vi "Mars3D_new.vi"(7 "Statemachine Data IN":T1={"Impulse Positions"=[], "Old Impulse positions for Undo"=[], "No. Imp"=0, "Parameter Time Series"=[], "Parameter Impuls Series"=[], "Experiment Parameters"={"Freq"=0.0, "Vel"=0, "Acc"=0, "Stimulus"=""}, "Autosort File"=refnum, "Data File"={"Data Channels"=[], "Sample Rate"=0, "Channel List"=[]}, "Experiment data path"=path "/Macintosh HD/Users/patrick/Studium/Diploma Thesis/Data Analysis", "Image data path"=path "/Macintosh HD/Users/patrick/Studium/Diploma Thesis/Data Analysis", "LVS data path"=path "/Macintosh HD/Users/patrick/Studium/Diploma Thesis/Data Analysis", "Raw copy path"=path "/Macintosh HD/Users/patrick/Studium/Diploma Thesis/Data Analysis", "filename"="No file selected", "desaccading parameters"={"Tolerance"=0, "Acc Range"=0.0, "Sample Rate"=0, "Impulse Plane 2"=enum."Other", "Impulse dir"=FALSE}, "Experiment Parameters 2"={"Subject"="", "Strain"="", "Rotation plane"="", "Experimenter"="", "Trial"=0.0, "Time"=0.0}, "Excel"={"Excel._Application"=refnum, "Use Excel"=FALSE, "Worksheet SINE"=refnum, "Row SINE"=0, "Worksheet TRANS"=refnum, "Row TRANS"=0}, "Session Config File"=refnum, "Autosort Parameter Set"=1, "EMA Version"="", "desacc "={"Threshold 1 [Acc]"=1617.080808080808, "Threshold 2 [% of TH1]"=67, "tolerance"=5, "Search WD "=0.19090909090909092, " always use TH2"=TRUE, "Range"=3.2323232323232323, "Max time"=200.0, "Min time"=20.0, "Velocity Threshold"=67}, "Cycle Nr for Saccades"={"POS"=0, "NEG"=0}, "Undo Counter"=0, "History Length"=0, "Redo Counter"=0, "Histpry Position"=0, "Raw Data File"={"Data Channels"=[], "Sample Rate"=0, "Channel List"=[]}, "calibration name"="No file selected"} {"Parameter Time Series"."time offset" format="%.3f"; "Parameter Time Series"."Gain" format="%.1f"; "Parameter Time Series"."Offset" format="%.1f"; "Parameter Time Series"."List 1" items=["Motor-Pos", "Motor-Vel", "Lx Position-in-Head", "Ly Position-in-Head", "Lz Position-in-Head", "Lx Velocity-in-Head", "Ly Velocity-in-Head", "Lz Velocity-in-Head", "Ll Velocity-in-Head", "Lr Velocity-in-Head", "Lx Accel-in-Head", "Ly Accel-in-Head", "Lz Accel-in-Head", "Rx Position-in-Head", "Ry Position-in-Head", "Rz Position-in-Head", "Rx Velocity-in-Head", "Ry Velocity-in-Head", "Rz Velocity-in-Head", "Rl Velocity-in-Head", "Rr Velocity-in-Head", "Rx Accel-in-Head", "Ry Accel-in-Head", "Rz Accel-in-Head", "Global Trigger", "", "", ""]; "Parameter Impuls Series"."Gain" format="%.1f"; "Parameter Impuls Series"."Offset" format="%.1f"}, 10 "File":path) -> (1 "stop 3":bool, 5 "Statemachine Data OUT":T1={"Impulse Positions"=[], "Old Impulse positions for Undo"=[], "No. Imp"=0, "Parameter Time Series"=[], "Parameter Impuls Series"=[], "Experiment Parameters"={"Freq"=0.0, "Vel"=0, "Acc"=0, "Stimulus"=""}, "Autosort File"=refnum, "Data File"={"Data Channels"=[], "Sample Rate"=0, "Channel List"=[]}, "Experiment data path"=path "/Macintosh HD/Users/patrick/Studium/Diploma Thesis/Data Analysis", "Image data path"=path "/Macintosh HD/Users/patrick/Studium/Diploma Thesis/Data Analysis", "LVS data path"=path "/Macintosh HD/Users/patrick/Studium/Diploma Thesis/Data Analysis", "Raw copy path"=path "/Macintosh HD/Users/patrick/Studium/Diploma Thesis/Data Analysis", "filename"="No file selected", "desaccading parameters"={"Tolerance"=0, "Acc Range"=0.0, "Sample Rate"=0, "Impulse Plane 2"=enum."Other", "Impulse dir"=FALSE}, "Experiment Parameters 2"={"Subject"="", "Strain"="", "Rotation plane"="", "Experimenter"="", "Trial"=0.0, "Time"=0.0}, "Excel"={"Excel._Application"=refnum, "Use Excel"=FALSE, "Worksheet SINE"=refnum, "Row SINE"=0, "Worksheet TRANS"=refnum, "Row TRANS"=0}, "Session Config File"=refnum, "Autosort Parameter Set"=1, "EMA Version"="", "desacc "={"Threshold 1 [Acc]"=1617.080808080808, "Threshold 2 [% of TH1]"=67, "tolerance"=5, "Search WD "=0.19090909090909092, " always use TH2"=TRUE, "Range"=3.2323232323232323, "Max time"=200.0, "Min time"=20.0, "Velocity Threshold"=67}, "Cycle Nr for Saccades"={"POS"=0, "NEG"=0}, "Undo Counter"=0, "History Length"=0, "Redo Counter"=0, "Histpry Position"=0, "Raw Data File"={"Data Channels"=[], "Sample Rate"=0, "Channel List"=[]}, "calibration name"="No file selected"} {"Parameter Time Series"."time offset" format="%.3f"; "Parameter Time Series"."Gain" format="%.1f"; "Parameter Time Series"."Offset" format="%.1f"; "Parameter Time Series"."List 1" items=["Motor-Pos", "Motor-Vel", "Lx Position-in-Head", "Ly Position-in-Head", "Lz Position-in-Head", "Lx Velocity-in-Head", "Ly Velocity-in-Head", "Lz Velocity-in-Head", "Ll Velocity-in-Head", "Lr Velocity-in-Head", "Lx Accel-in-Head", "Ly Accel-in-Head", "Lz Accel-in-Head", "Rx Position-in-Head", "Ry Position-in-Head", "Rz Position-in-Head", "Rx Velocity-in-Head", "Ry Velocity-in-Head", "Rz Velocity-in-Head", "Rl Velocity-in-Head", "Rr Velocity-in-Head", "Rx Accel-in-Head", "Ry Accel-in-Head", "Rz Accel-in-Head", "Global Trigger", "", "", ""]; "Parameter Impuls Series"."Gain" format="%.1f"; "Parameter Impuls Series"."Offset" format="%.1f"})   [LabVIEW 2016]
uses:
  core/type-defs/TD_Statemachine-Data.ctl
  core/type-defs/TD_Time Series.ctl
  core/type-defs/TD_Impulse Parameter.ctl
  <vilib>/Utility/file.llb/Read From Spreadsheet File (DBL).vi
  tracking algorithmus/3 dot tracker.lvlib
  <vilib>/Analysis/NI_AALPro.lvlib
  core/core.lvlib
panel:
  in  "Savol Filter in percent":dbl=3.0 format="%#_13g"
  in  "stop 2":bool
  in  "VOG system":enum16{"Mouse", "Chinchilla"}(ring)
  in  "Tab Control":T4(tab)
  in  "Savgol":bool
  in  "Right Eye":T5 {"y" format="%.2f"; "z" format="%.2f"; "theta" format="%.2f"; "phi" format="%.2f"; "d" format="%.2f"}
  in  "Left Eye":T5 {"y" format="%.2f"; "z" format="%.2f"; "theta" format="%.2f"; "phi" format="%.2f"; "d" format="%.2f"}
  in  "Position Convention":u16(ring)=1 items=["Fick Angles", "Rotation Vectors"]
  in  "Angles":bool
  in  "Automatic Calibration":bool=TRUE
  in  "Rev Cam?":bool caption="Reverse Camera\nOrientation?"
  in  "Plot Selection":T2=[{"time offset"=0.0, "Offset"=0.0, "Gain"=1.0, "inverse"=FALSE, "filter data"=FALSE, "dots"=FALSE, "interpolate"=FALSE, "List 1"=1, "Color Box"=0, "Boolean"=TRUE}, {"time offset"=0.0, "Offset"=0.0, "Gain"=1.0, "inverse"=FALSE, "filter data"=FALSE, "dots"=FALSE, "interpolate"=FALSE, "List 1"=7, "Color Box"=16860, "Boolean"=TRUE}, {"time offset"=0.0, "Offset"=0.0, "Gain"=1.0, "inverse"=FALSE, "filter data"=FALSE, "dots"=FALSE, "interpolate"=FALSE, "List 1"=18, "Color Box"=16711680, "Boolean"=TRUE}] {"time offset" format="%.3f"; "Gain" format="%.1f"; "Offset" format="%.1f"; "List 1" items=["Motor-Pos", "Motor-Vel", "Lx Position-in-Head", "Ly Position-in-Head", "Lz Position-in-Head", "Lx Velocity-in-Head", "Ly Velocity-in-Head", "Lz Velocity-in-Head", "Ll Velocity-in-Head", "Lr Velocity-in-Head", "Lx Accel-in-Head", "Ly Accel-in-Head", "Lz Accel-in-Head", "Rx Position-in-Head", "Ry Position-in-Head", "Rz Position-in-Head", "Rx Velocity-in-Head", "Ry Velocity-in-Head", "Rz Velocity-in-Head", "Rl Velocity-in-Head", "Rr Velocity-in-Head", "Rx Accel-in-Head", "Ry Accel-in-Head", "Rz Accel-in-Head", "Global Trigger", "Free 1", "Free 2", "Free 3"]}
  in  "Plot Selection 2":T3=[{"Color"=4652800, "Visible"=TRUE, "Channel"=1, "Invert"=FALSE, "Desaccade"=FALSE, "Offset"=0.0, "Gain"=1.0}, {"Color"=16860, "Visible"=TRUE, "Channel"=7, "Invert"=FALSE, "Desaccade"=FALSE, "Offset"=0.0, "Gain"=1.0}, {"Color"=16711680, "Visible"=TRUE, "Channel"=18, "Invert"=FALSE, "Desaccade"=FALSE, "Offset"=0.0, "Gain"=1.0}] {"Gain" format="%.1f"; "Offset" format="%.1f"; "Channel" items=["Motor-Pos", "Motor-Vel", "Lx Position-in-Head", "Ly Position-in-Head", "Lz Position-in-Head", "Lx Velocity-in-Head", "Ly Velocity-in-Head", "Lz Velocity-in-Head", "Ll Velocity-in-Head", "Lr Velocity-in-Head", "Lx Accel-in-Head", "Ly Accel-in-Head", "Lz Accel-in-Head", "Rx Position-in-Head", "Ry Position-in-Head", "Rz Position-in-Head", "Rx Velocity-in-Head", "Ry Velocity-in-Head", "Rz Velocity-in-Head", "Rl Velocity-in-Head", "Rr Velocity-in-Head", "Rx Accel-in-Head", "Ry Accel-in-Head", "Rz Accel-in-Head", "Global Trigger", "Free 1", "Free 2", "Free 3"]}
  in  "Tolerance":i32(slide)=40 step=2 scale=0.0..100.0
  in  "Acc Range":dbl(slide)=3000.0 step=50.0 scale=0.0..30000.0
  in  "Impulse dir":bool
  in  "Impulse Plane 2":T6(ring)=enum."Yaw" caption="Impulse Plane"
  in  "process":bool
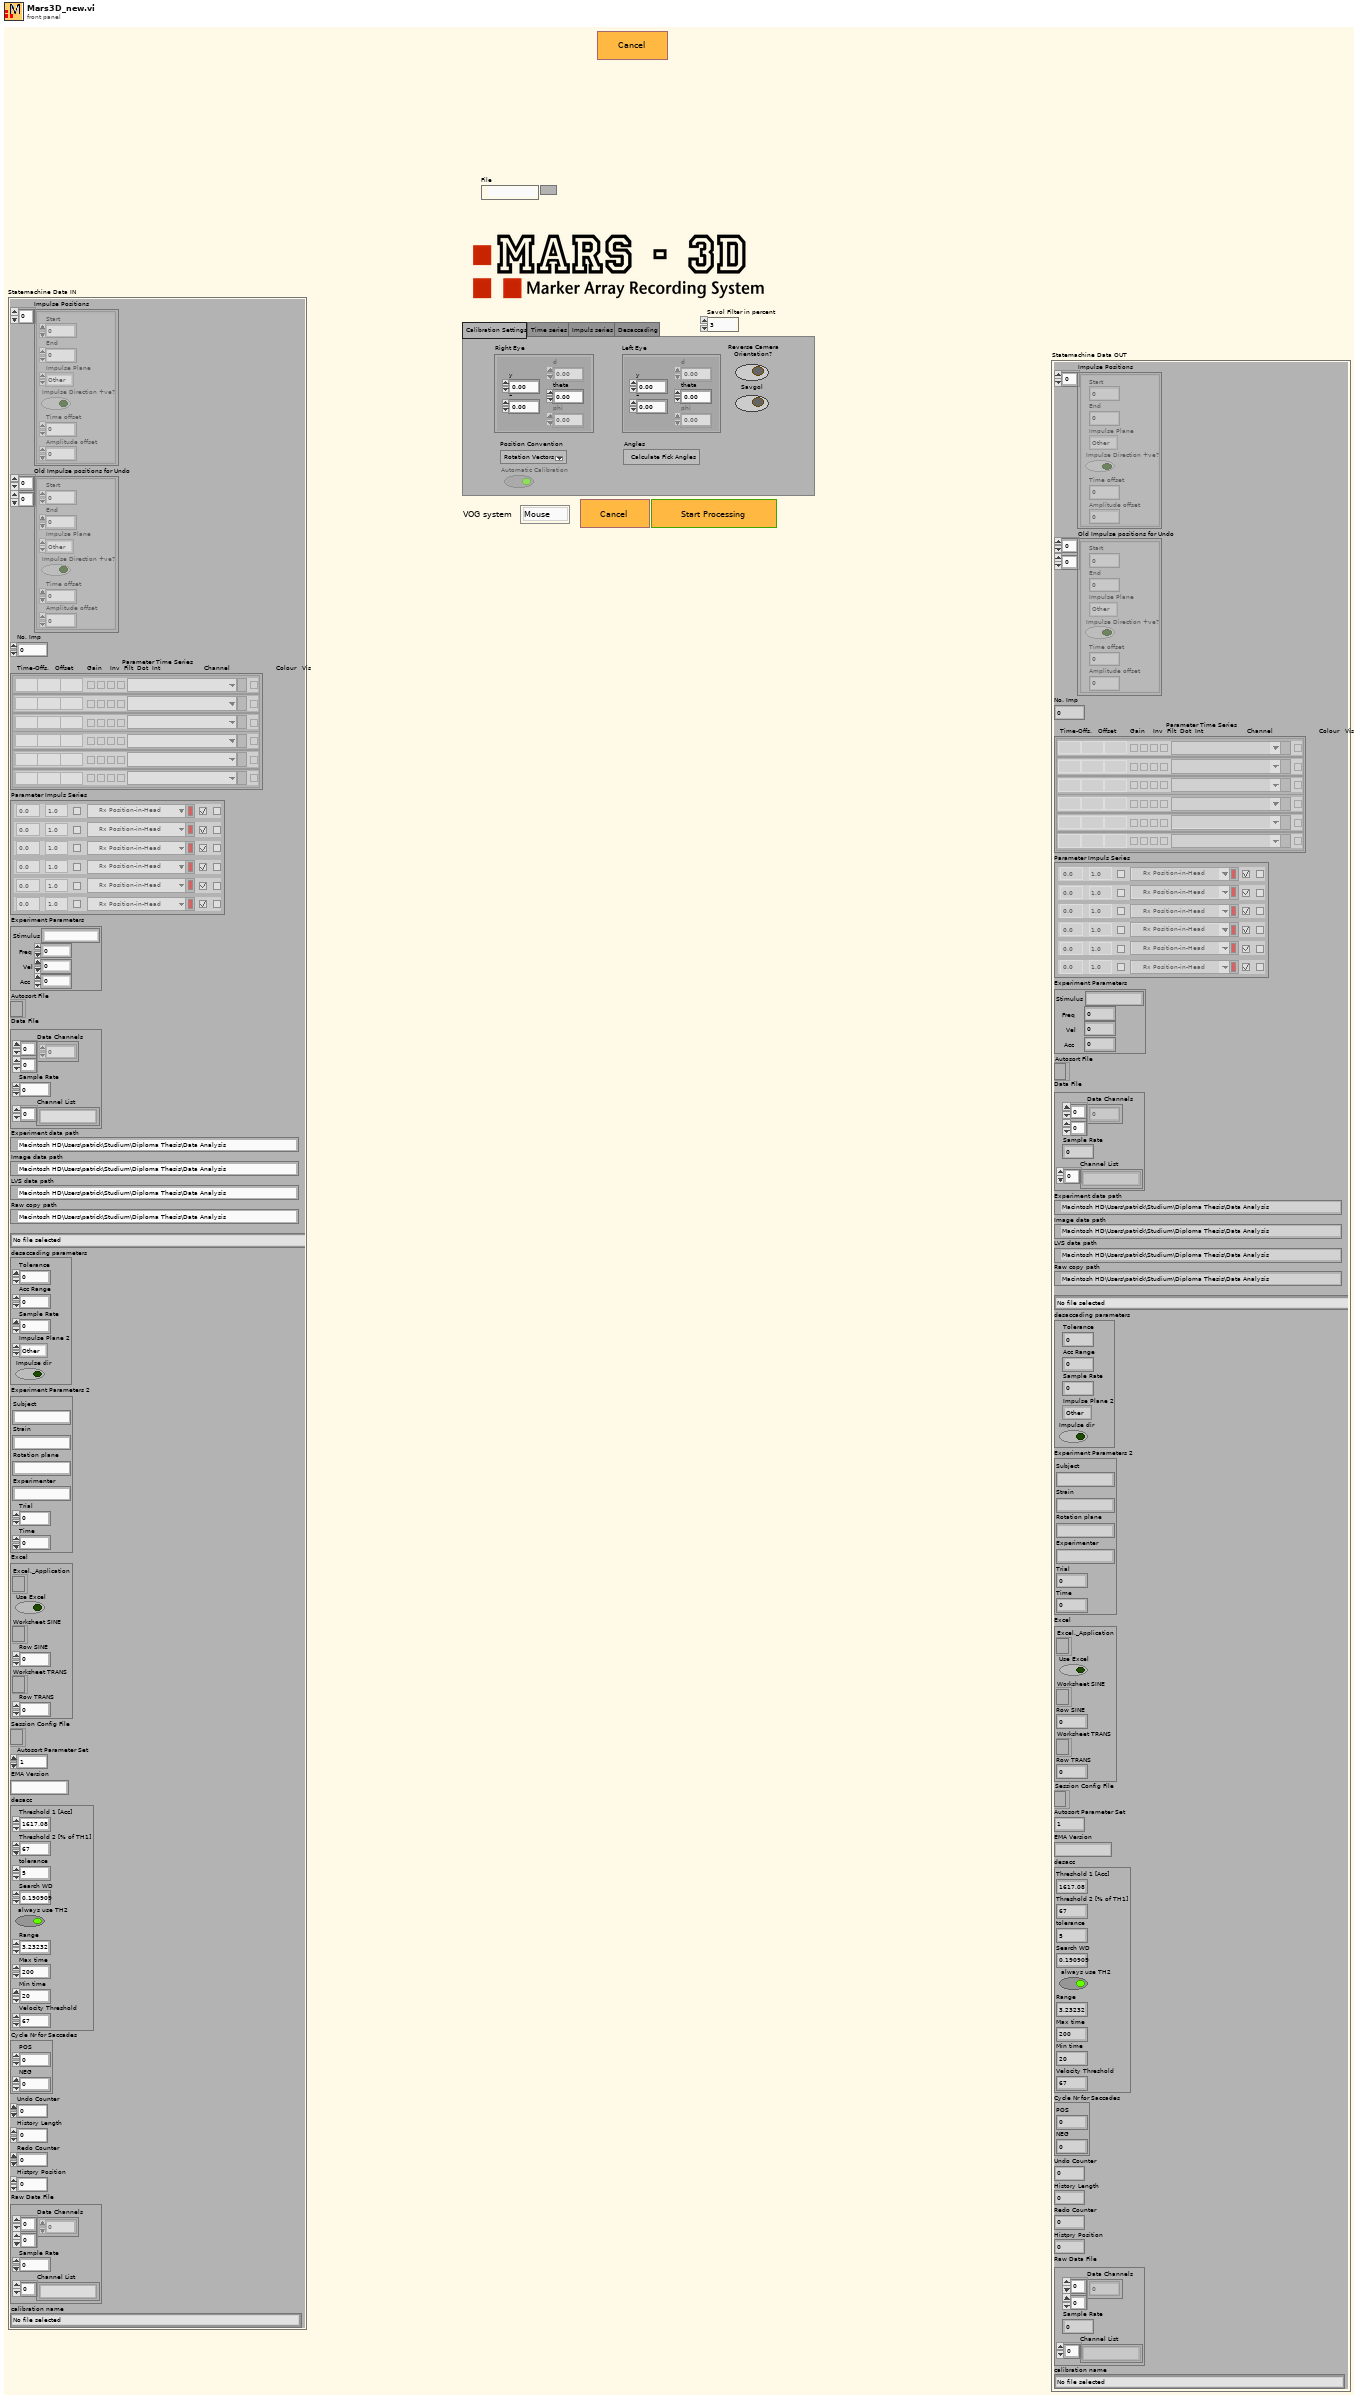
[diagram p1: front panel]
types:
  T1 = typedef "core.lvlib/TD_Statemachine-Data.ctl" = cluster{"Impulse Positions":cluster{"Start":i32, "End":i32, "Impulse Plane":enum16{"Other", "Yaw", "Pitch", "Roll", "LARP", "RALP"}, "Impulse Direction +ve?":bool, "Time offset":i32, "Amplitude offset":dbl}[], "Old Impulse positions for Undo":cluster{"Start":i32, "End":i32, "Impulse Plane":enum16{"Other", "Yaw", "Pitch", "Roll", "LARP", "RALP"}, "Impulse Direction +ve?":bool, "Time offset":i32, "Amplitude offset":dbl}[][], "No. Imp":i32, "Parameter Time Series":T2, "Parameter Impuls Series":T3, "Experiment Parameters":cluster{"Freq":dbl, "Vel":i32, "Acc":i32, "Stimulus":string}, "Autosort File":refnum<file>, "Data File":cluster{"Data Channels":dbl[][], "Sample Rate":i32, "Channel List":string[]}, "Experiment data path":path, "Image data path":path, "LVS data path":path, "Raw copy path":path, "filename":string, "desaccading parameters":cluster{"Tolerance":i32, "Acc Range":dbl, "Sample Rate":i32, "Impulse Plane 2":enum16{"Other", "Yaw", "Pitch", "Roll", "LARP", "RALP"}, "Impulse dir":bool}, "Experiment Parameters 2":cluster{"Subject":string, "Strain":string, "Rotation plane":string, "Experimenter":string, "Trial":dbl, "Time":dbl}, "Excel":cluster{"Excel._Application":refnum<k7>, "Use Excel":bool, "Worksheet SINE":refnum<k7>, "Row SINE":i32, "Worksheet TRANS":refnum<k7>, "Row TRANS":i32}, "Session Config File":refnum<file>, "Autosort Parameter Set":i32, "EMA Version":string, "desacc ":cluster{"Threshold 1 [Acc]":dbl, "Threshold 2 [% of TH1]":i32, "tolerance":i32, "Search WD ":dbl, " always use TH2":bool, "Range":dbl, "Max time":dbl, "Min time":dbl, "Velocity Threshold":i32}, "Cycle Nr for Saccades":cluster{"POS":i32, "NEG":i32}, "Undo Counter":i32, "History Length":i32, "Redo Counter":i32, "Histpry Position":i32, "Raw Data File":cluster{"Data Channels":dbl[][], "Sample Rate":i32, "Channel List":string[]}, "calibration name":string}
  T2 = typedef "core.lvlib/TD_Time Series.ctl" = cluster{"time offset":dbl, "Offset":dbl, "Gain":dbl, "inverse":bool, "filter data":bool, "dots":bool, "interpolate":bool, "List 1":u16, "Color Box":u32, "Boolean":bool}[]
  T3 = typedef "core.lvlib/TD_Impulse Parameter.ctl" = cluster{"Color":u32, "Visible":bool, "Channel":u16, "Invert":bool, "Desaccade":bool, "Offset":dbl, "Gain":dbl}[]
  T4 = enum32{"Calibration Settings", "Time series", "Impuls series", "Desaccading"}
  T5 = cluster{"d":dbl, "phi":dbl, "theta":dbl, "z":dbl, "y":dbl}
  T6 = enum16{"Other", "Yaw", "Pitch", "Roll", "LARP", "RALP"}
  T7 = cluster{"Tolerance":i32, "Acc Range":dbl, "Sample Rate":i32, "Impulse Plane 2":enum16{"Other", "Yaw", "Pitch", "Roll", "LARP", "RALP"}, "Impulse dir":bool}
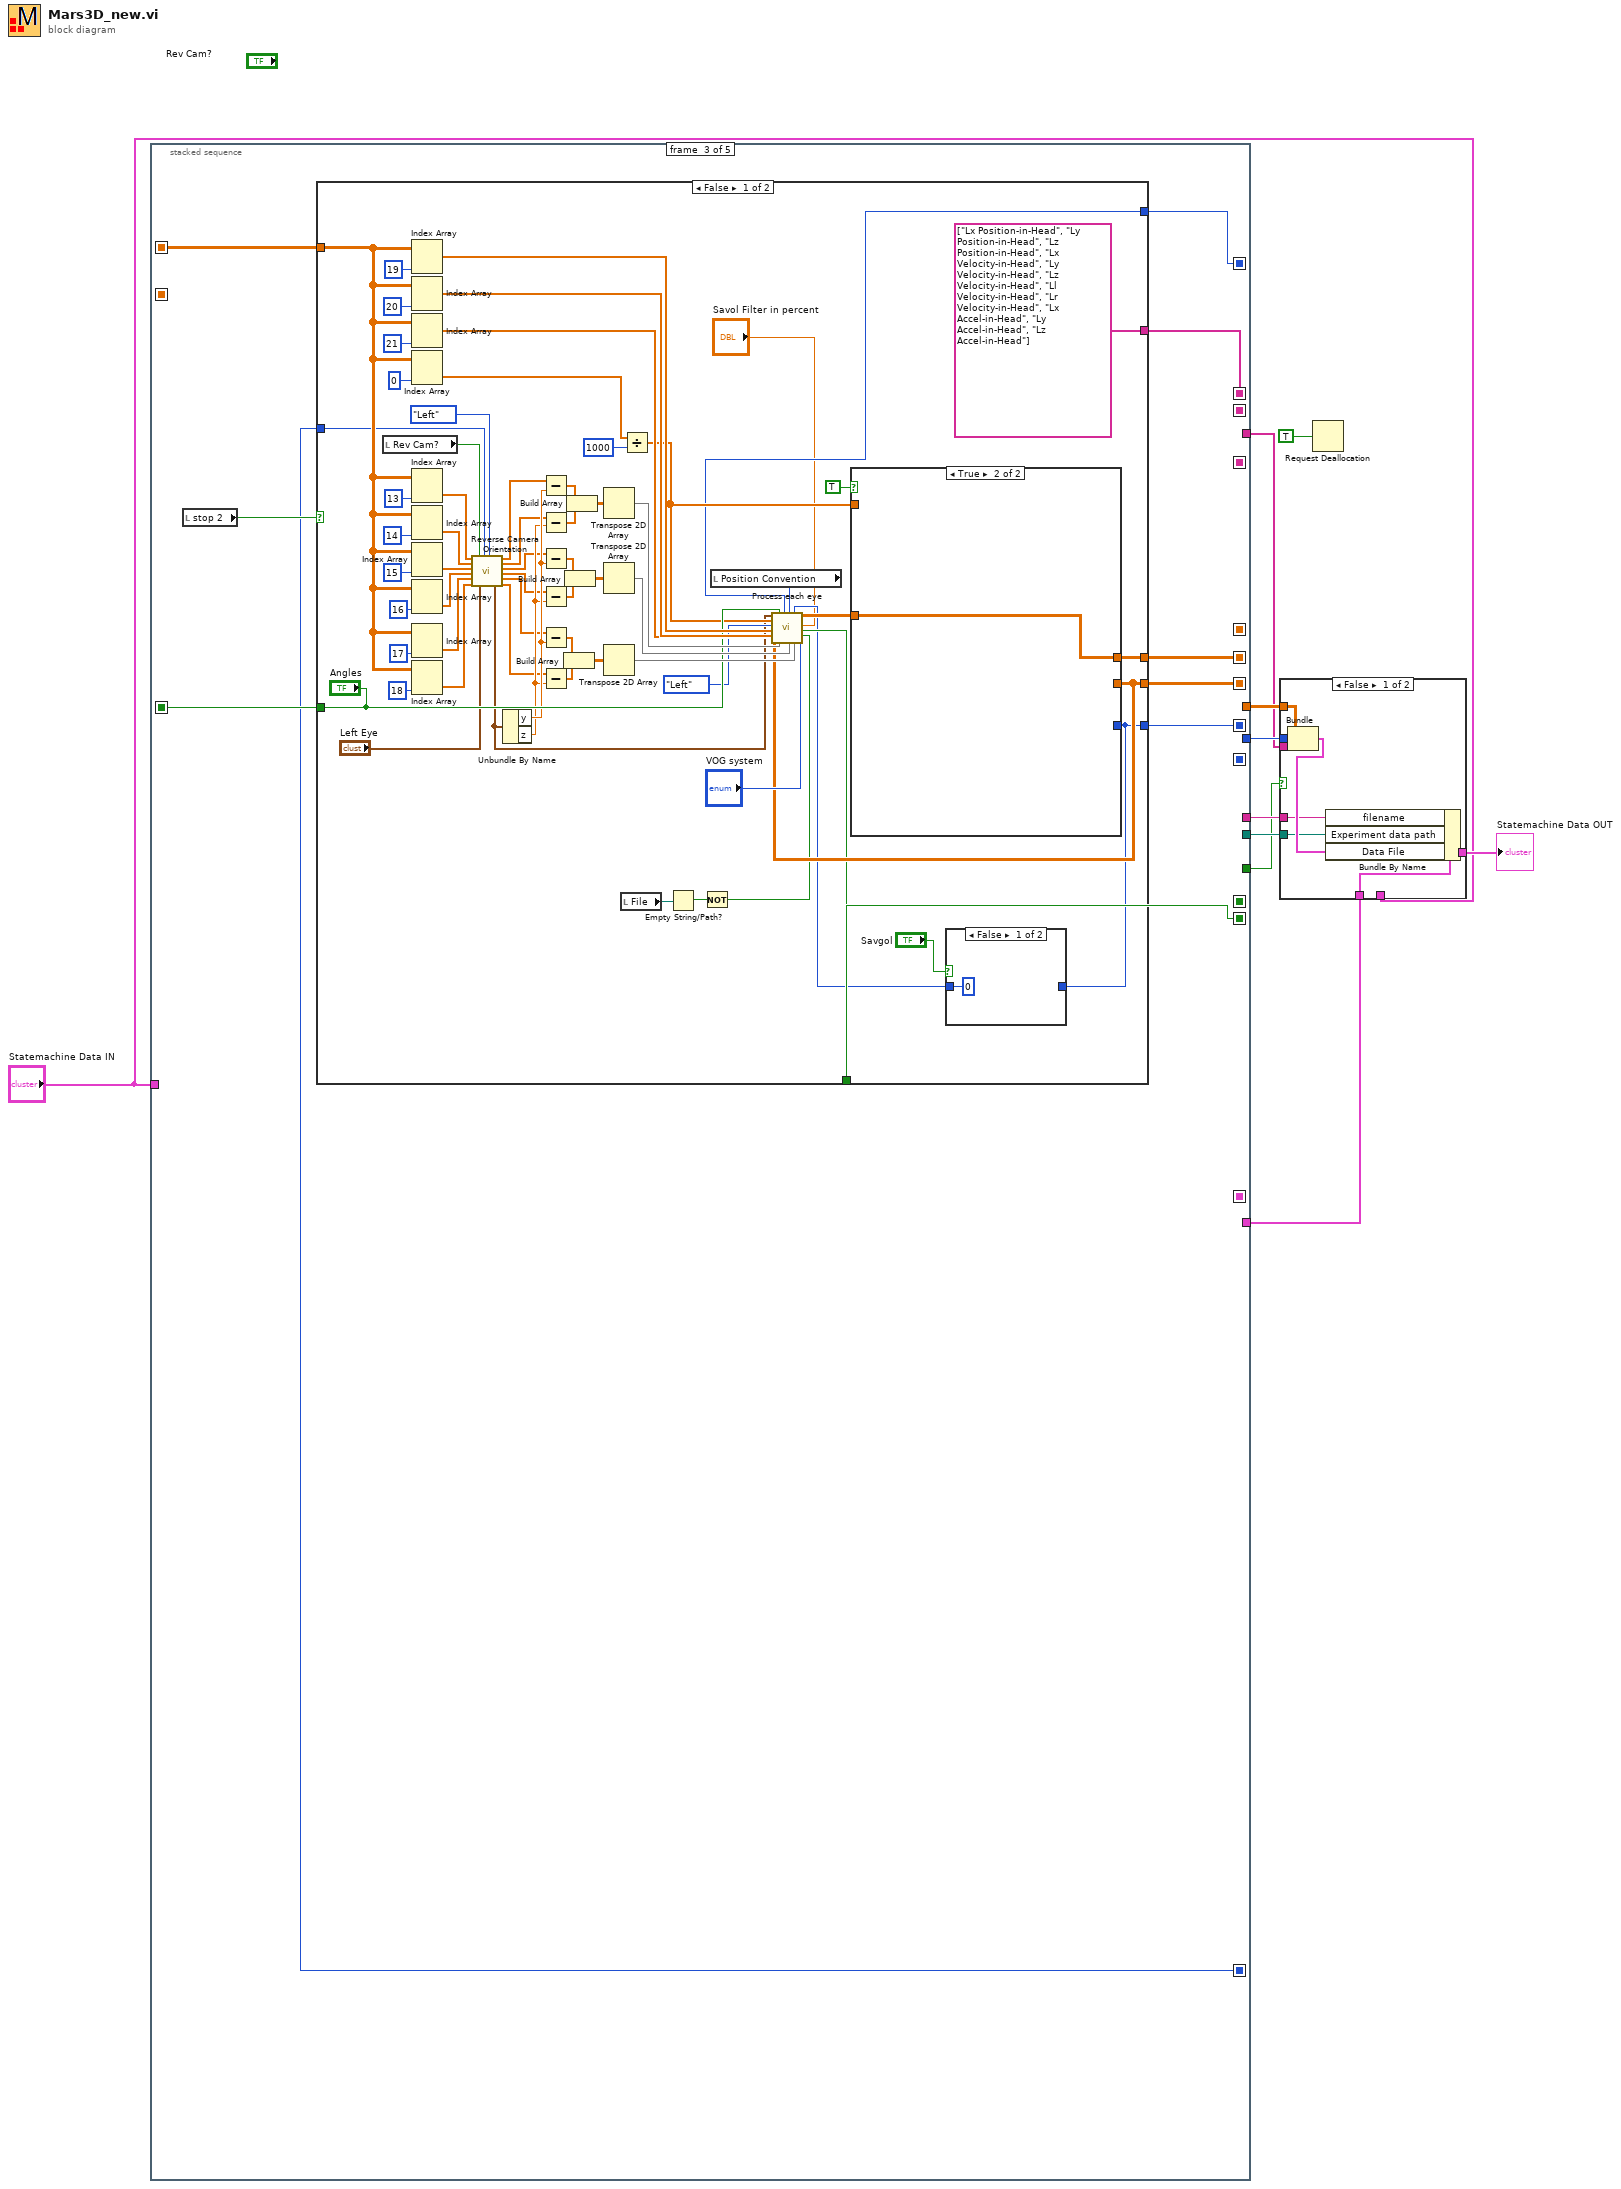
[diagram p0: block diagram]
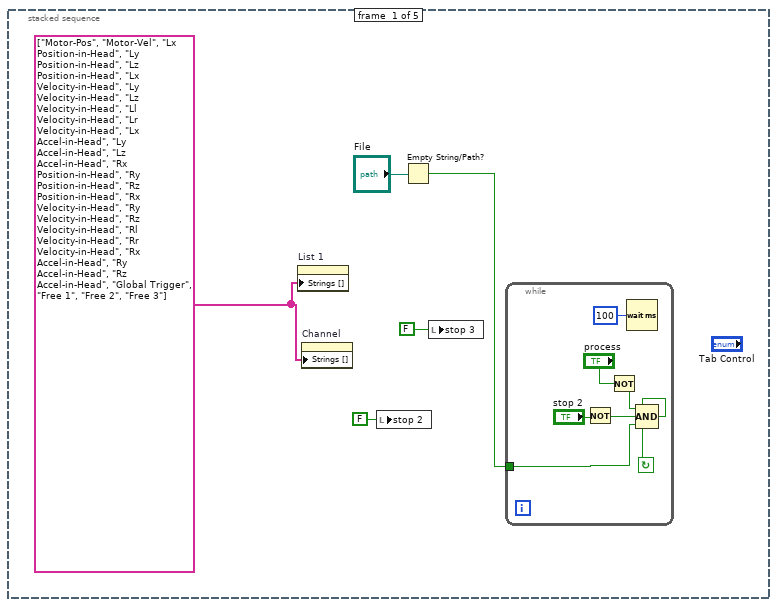
[diagram p3: hidden frame]
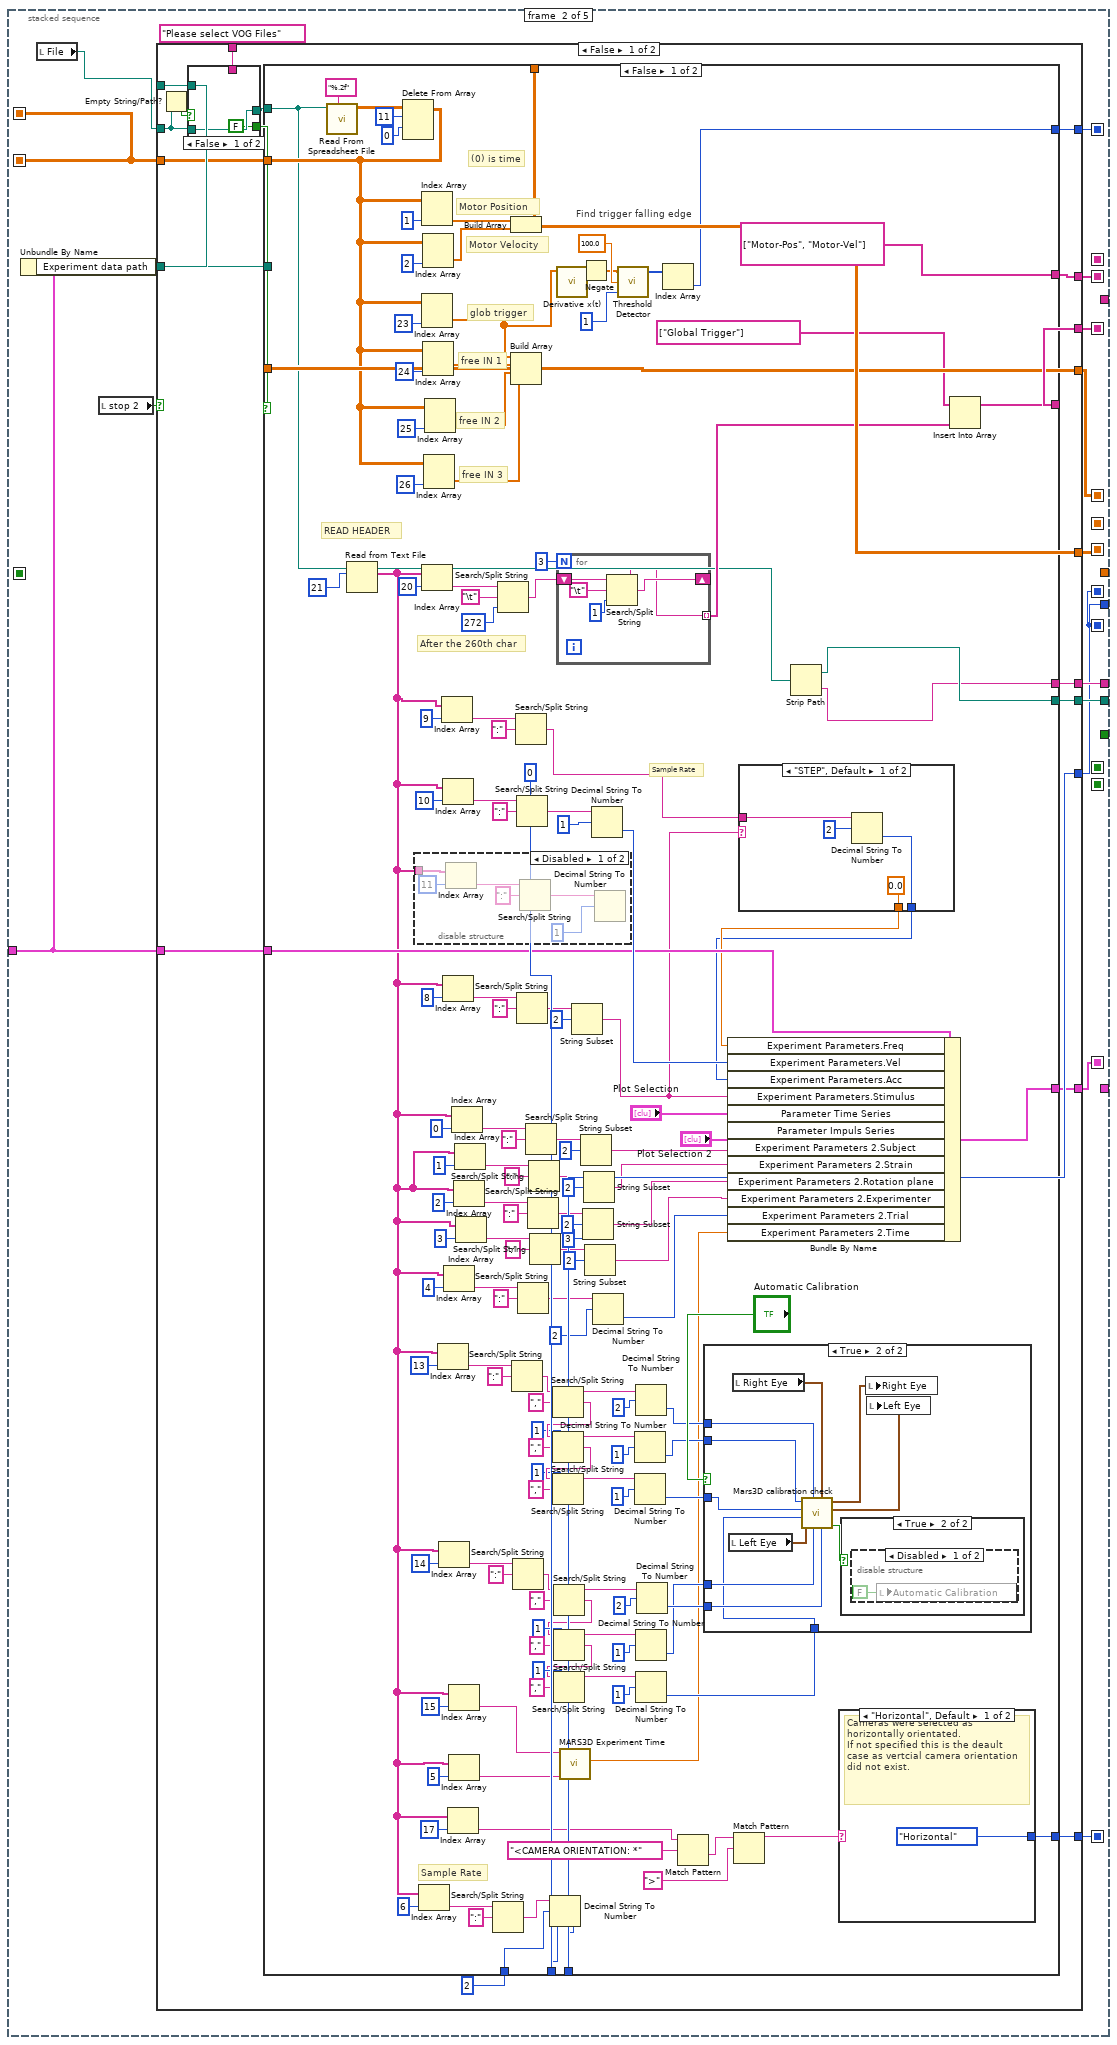
[diagram p4: hidden frame]
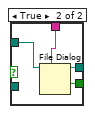
[diagram p5: hidden frame]
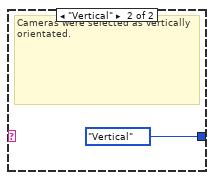
[diagram p6: hidden frame]
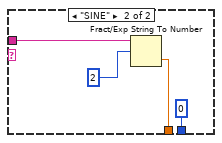
[diagram p7: hidden frame]
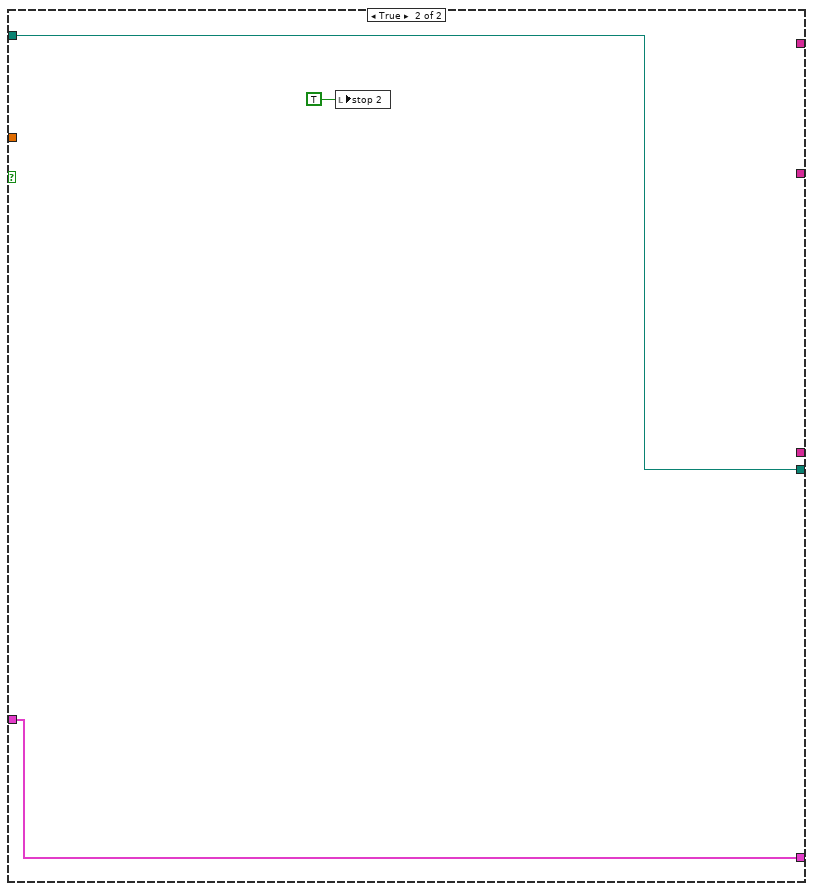
[diagram p12: hidden frame]
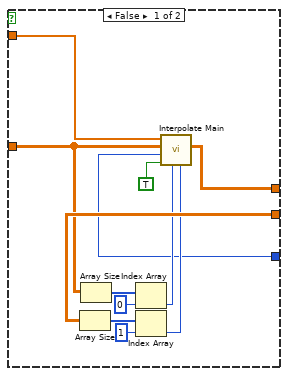
[diagram p15: hidden frame]
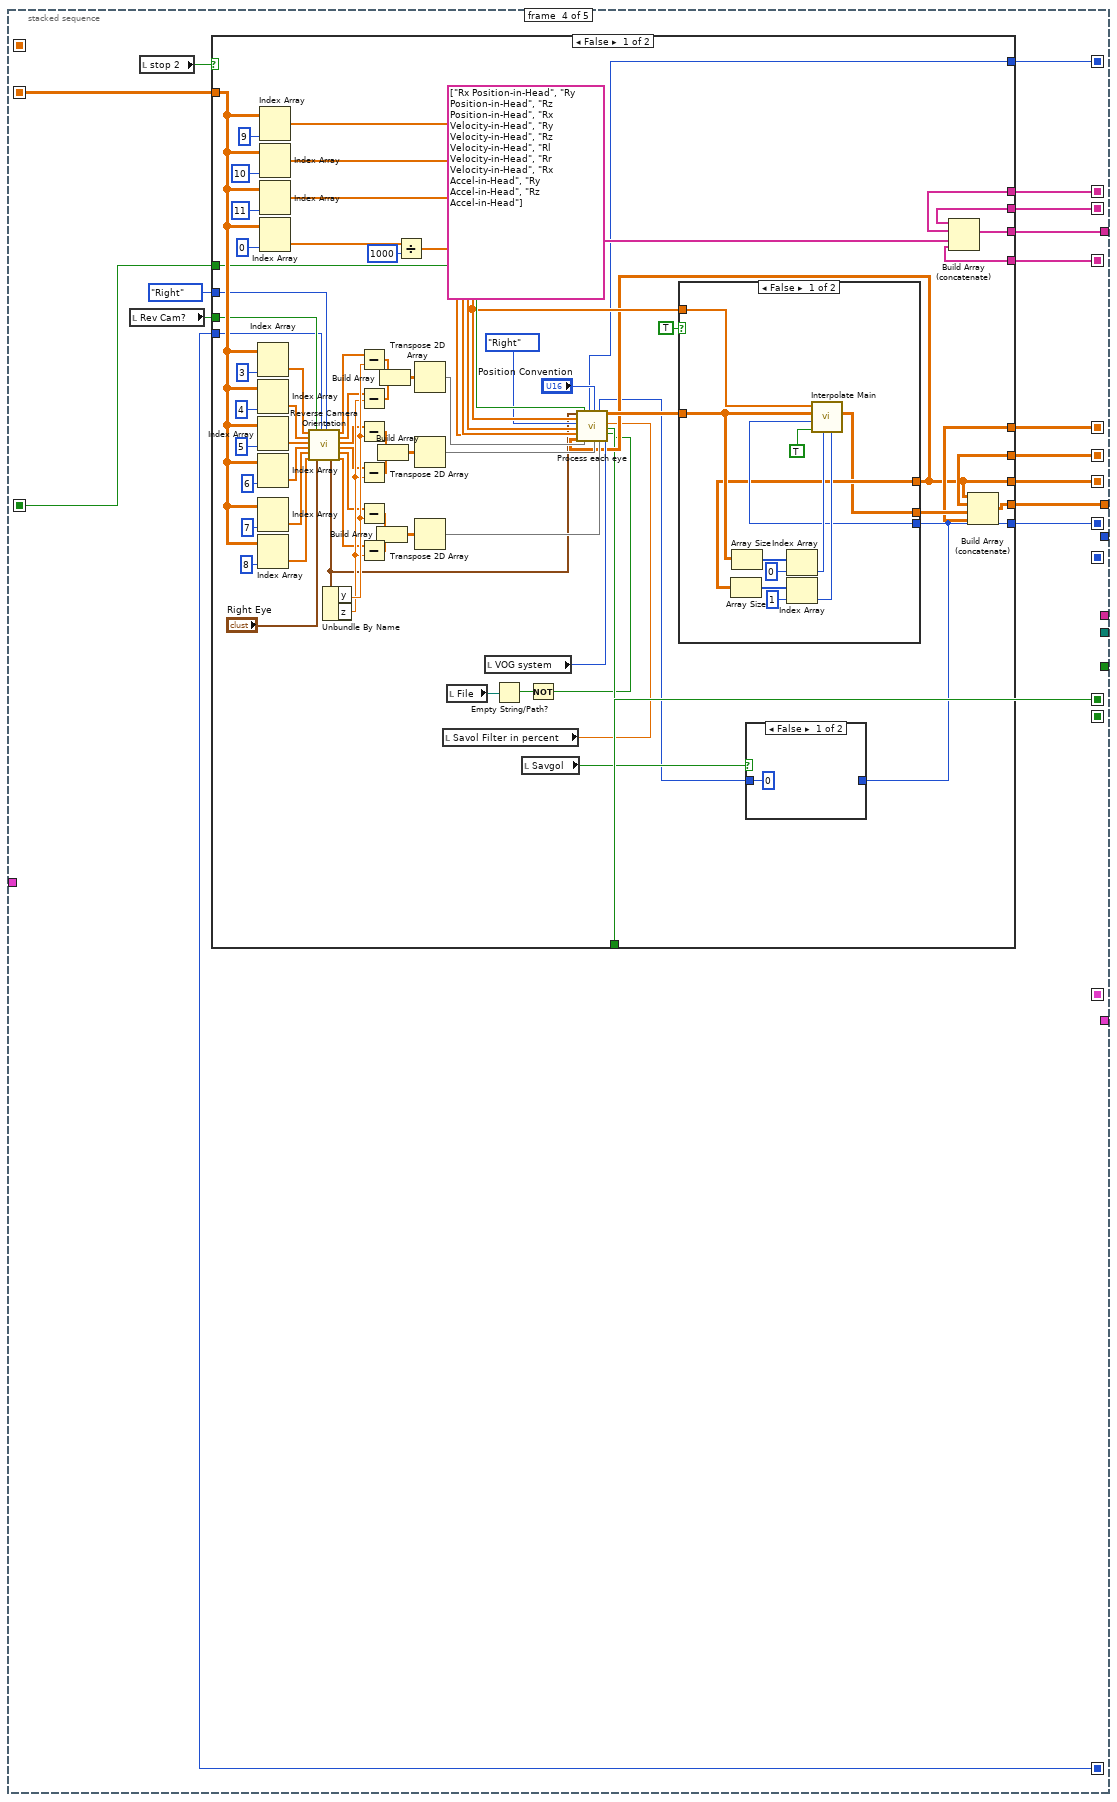
[diagram p17: hidden frame]
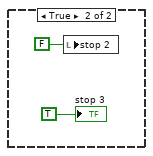
[diagram p20: hidden frame]
diagram:
  n1 = stacked-sequence {
    seq-local: [_ w38 _ _ _] -> [_ _ _ w362 _]
    seq-local: [_ w37 _ _ _] -> [_ _ w264 w356 _]
    seq-local: [_ w27 _ _ _] -> [_ _ w263 w357 _]
    seq-local: [_ w36 _ _ _] -> [_ _ _ w364 _]
    seq-local: [_ _ w266 _ _] -> [_ _ _ w363 _]
    seq-local: [_ _ w265 _ _] -> [_ _ _ w361 _]
    seq-local: [_ _ w262 _ _] -> [_ _ _ w358 _]
    seq-local: [_ w36 _ _ _] -> [_ _ w261 _ _]
    seq-local: [_ w35 _ _ _] -> [_ _ _ w354 _]
    seq-local: [_ w34 _ _ _] -> [_ _ _ w355 _]
    seq-local: [_ w27 _ _ _] -> [_ _ _ _ w465]
    seq-local: [_ w26 _ _ _] -> [_ _ _ _ w463]
    seq-local: [_ w25 _ _ _] -> [_ _ w259 w352 _]
    seq-local: [_ _ w258 _ _] -> [_ _ _ _ w458]
    seq-local: [_ _ _ w351 _] -> [_ _ _ _ w459]
    seq-local: [_ w23 _ _ _] -> [_ _ w257 w350 _]
    tunnel: [_ _ _ w360 _] -> w9
    tunnel: [_ _ _ w359 _] -> w7
    tunnel: [_ w27 _ _ _] -> w10
    tunnel: [_ _ _ _ w461] -> w6
    tunnel: "Statemachine Data IN" -> [_ w31 _ _ _]
    tunnel: [_ w30 _ _ _] -> w4
    tunnel: [_ w28 _ _ _] -> w3
    tunnel: [_ _ _ _ w456] -> w1
    frame #0 {
      w14 = string[] ["Motor-Pos", "Motor-Vel", "Lx Position-in-Head", "Ly Position-in-Head", "Lz Position-in-Head", "Lx Velocity-in-Head", "Ly Velocity-in-Head", "Lz Velocity-in-Head", "Ll Velocity-in-Head", "Lr Velocity-in-Head", "Lx Accel-in-Head", "Ly Accel-in-Head", "Lz Accel-in-Head", "Rx Position-in-Head", "Ry Position-in-Head", "Rz Position-in-Head", "Rx Velocity-in-Head", "Ry Velocity-in-Head", "Rz Velocity-in-Head", "Rl Velocity-in-Head", "Rr Velocity-in-Head", "Rx Accel-in-Head", "Ry Accel-in-Head", "Rz Accel-in-Head", "Global Trigger", "Free 1", "Free 2", "Free 3"] ("Channel List")
      n2 = property on="List 1" class="Ring (strict)"("Strings []"=w14) -> ()  [unwired: 2 in, 2 out]
      n3 = property on="Channel" class="Ring (strict)"("Strings []"=w14) -> ()  [unwired: 2 in, 2 out]
      n4 = local write "stop 2"(FALSE ("stop 2")) -> ()
      n5 = Empty String/Path?(string/path="File") -> (empty?=w12:bool)
      n6 = local write "stop 3"(FALSE ("stop 3")) -> ()
      n7 = while {
        tunnel: w12 -> [w16]
        stop <- w17 continue-if-true
        n8 = Not(x="stop 2") -> (.not. x?=w19:bool)
        n9 = Not(x="process") -> (.not. x?=w18:bool)
        n10 = Wait (ms)(milliseconds to wait=u32 100) -> ()  [unwired: 1 out]
        n11 = Compound Arithmetic op=AND(w18, w19, w16) -> (w17:bool)
      }
    }
    frame #1 {
      (unwired) 0 ("ADD1")
      (unwired) 0 ("ADD1")
      (unwired) 0 ("ADD1")
      n12 = Unbundle By Name(w31) -> ("Experiment data path"=w29:path)
      n13 = local read "File"() -> (w24:path)
      n14 = local read "stop 2"() -> (w33:bool)
      n15 = case shown="False" w33 {
        tunnel: [w59 _] -> w38
        tunnel: [w58 _] -> w37
        tunnel: [w56 _] -> w27
        tunnel: [w55 _] -> w36
        tunnel: [w54 _] -> w35
        tunnel: [w53 _] -> w34
        tunnel: "Please select VOG Files" ("prompt") -> [w50 _]
        tunnel: w29 -> [w48 w255]
        tunnel: [w47 w256] -> w26
        tunnel: w31 -> [w46 w256]
        tunnel: [w45 w255] -> w30
        tunnel: w29 -> [w44 _]
        tunnel: [w43 _] -> w28
        tunnel: [w42 _] -> w25
        tunnel: w24 -> [w41 _]
        tunnel: [w39 _] -> w23
        frame False {
          # "Sample Rate"
          n16 = Empty String/Path?(string/path=w41) -> (empty?=w40:bool)
          n17 = case shown="False" w40 {
            tunnel: [w61 w65] -> w51
            tunnel: w50 -> [_ w64]
            tunnel: [FALSE ("cancelled") w63] -> w49
            tunnel: w48 -> [_ w62]
            tunnel: w41 -> [w61 _]
            frame False {
            }
            frame True {
              n18 = File Dialog(7:w64, 11:w62) -> (1:w63:bool, 3:w65:path)  [unwired: 5 in, 2 out]
            }
          }
          n19 = case shown="False" w49 {
            tunnel: [string[] ["Motor-Pos", "Motor-Vel"] _] -> w59
            tunnel: [w212 _] -> w58
            tunnel: 0 ("default (0 I32)") -> [w206 _]
            tunnel: [w205 _] -> w56
            tunnel: [w197 _] -> w55
            tunnel: [w189 _] -> w54
            tunnel: [w184 _] -> w53
            tunnel: 2 ("offset") -> [w183 _]
            tunnel: w51 -> [w182 _]
            tunnel: [w165 w253] -> w47
            tunnel: w46 -> [w164 w253]
            tunnel: [w163 w252] -> w45
            tunnel: w44 -> [_ w252]
            tunnel: [w162 _] -> w43
            tunnel: [w74 _] -> w42
            tunnel: [w66 _] -> w39
            frame False {
              # "READ HEADER"
              # "Find trigger falling edge"
              # "Sample Rate"
              # "free IN 3"
              # "free IN 2"
              # "free IN 1"
              # "glob trigger"
              # "After the 260th char"
              # "(0) is time"
              # "Motor Velocity"
              # "Motor Position"
              n20 = call-poly <vilib>:"Read From Spreadsheet File.vi"("format (%.3f)"="%.2f", "file path (dialog if empty)"=w182) -> ("all rows"=w204:dbl[][])  [unwired: 5 in, 4 out]
              n21 = Read from Text File(file (use dialog)=w182, count=21) -> (text=w73:string[])  [unwired: 2 in, 3 out]
              n22 = Delete From Array(array=w204, length=11, index (row)=0) -> (array with subset deleted=w197:dbl[][])  [unwired: 1 in, 1 out]
              n23 = disable-structure shown="Disabled" {
                disable-tunnel: w73 -> [w229 _]
                frame Disabled {
                  n24 = Index Array(array=w229, index=11) -> (element=w233:string)
                  n25 = Search/Split String(string=w233, search string/char (-)=":") -> (match + rest of string=w231:string)  [unwired: 1 in, 2 out]
                  n26 = Decimal String To Number(string=w231, offset=1) -> ()  [unwired: 1 in, 2 out]
                }
                frame Enabled {
                }
              }
              n27 = Index Array(array=w73, index=6) -> (element=w209:string)
              n28 = Index Array(array=w197, index (col)=1 ("disabled index (col)")) -> (element=w214:dbl[])  [unwired: 1 in]
              n29 = Index Array(array=w197, index (col)=23 ("disabled index (col)")) -> (element=w80:dbl[])  [unwired: 1 in]
              n30 = Index Array(array=w73, index=20) -> (element=w195:string)
              n31 = Index Array(array=w197, index (col)=2 ("disabled index (col)")) -> (element=w213:dbl[])  [unwired: 1 in]
              n32 = Index Array(array=w197, index (col)=24 ("disabled index (col)")) -> (element=w187:dbl[])  [unwired: 1 in]
              n33 = Index Array(array=w197, index (col)=26 ("disabled index (col)")) -> (element=w185:dbl[])  [unwired: 1 in]
              n34 = Index Array(array=w197, index (col)=25 ("disabled index (col)")) -> (element=w186:dbl[])  [unwired: 1 in]
              n35 = Index Array(array=w73, index=13) -> (element=w128:string)
              n36 = Index Array(array=w73, index=14) -> (element=w96:string)
              n37 = Index Array(array=w73, index=9) -> (element=w170:string)
              n38 = Index Array(array=w73, index=10) -> (element=w175:string)
              n39 = Index Array(array=w73, index=8) -> (element=w180:string)
              n40 = Index Array(array=w73, index=4) -> (element=w135:string)
              n41 = Index Array(array=w73, index=17) -> (element=w68:string)
              n42 = Index Array(array=w73, index=15) -> (element=w88:string)
              n43 = Index Array(array=w73, index=5) -> (element=w87:string)
              n44 = Index Array(array=w73, index=0) -> (element=w158:string)
              n45 = Index Array(array=w73, index=2) -> (element=w146:string)
              n46 = Index Array(array=w73, index=1) -> (element=w155:string)
              n47 = Index Array(array=w73, index=3) -> (element=w142:string)
              n48 = Search/Split String(string=w209, search string/char (-)=":") -> (match + rest of string=w207:string)  [unwired: 1 in, 2 out]
              n49 = Search/Split String(string=w195, search string/char (-)="\t", offset (0)=272) -> (match + rest of string=w192:string)  [unwired: 2 out]
              n50 = Build Array(w214, w213) -> (w212:dbl[][])
              n51 = Build Array(w80, w187, w186, w185) -> (w184:dbl[][])
              n52 = Search/Split String(string=w128, search string/char (-)=":") -> (match + rest of string=w126:string)  [unwired: 1 in, 2 out]
              n53 = Search/Split String(string=w96, search string/char (-)=":") -> (match + rest of string=w98:string)  [unwired: 1 in, 2 out]
              n54 = Search/Split String(string=w170, search string/char (-)=":") -> (match + rest of string=w83:string)  [unwired: 1 in, 2 out]
              n55 = Search/Split String(string=w175, search string/char (-)=":") -> (match + rest of string=w173:string)  [unwired: 1 in, 2 out]
              n56 = Search/Split String(string=w180, search string/char (-)=":") -> (match + rest of string=w178:string)  [unwired: 1 in, 2 out]
              n57 = Search/Split String(string=w135, search string/char (-)=":") -> (match + rest of string=w137:string)  [unwired: 1 in, 2 out]
              n58 = Search/Split String(string=w158, search string/char (-)=":") -> (match + rest of string=w160:string)  [unwired: 1 in, 2 out]
              n59 = Search/Split String(string=w146, search string/char (-)=":") -> (match + rest of string=w148:string)  [unwired: 1 in, 2 out]
              n60 = Search/Split String(string=w155, search string/char (-)=":") -> (match + rest of string=w153:string)  [unwired: 1 in, 2 out]
              n61 = Search/Split String(string=w142, search string/char (-)=":") -> (match + rest of string=w140:string)  [unwired: 1 in, 2 out]
              n62 = Decimal String To Number(string=w207, offset=w183, default (0L)=w206) -> (number=w205:i32)  [unwired: 1 out]
              n63 = Search/Split String(string=w126, search string/char (-)=",") -> (substring before match=w124:string, match + rest of string=w122:string)  [unwired: 1 in, 1 out]
              n64 = Search/Split String(string=w122, search string/char (-)=",", offset (0)=1) -> (substring before match=w120:string, match + rest of string=w116:string)  [unwired: 1 out]
              n65 = Search/Split String(string=w116, search string/char (-)=",", offset (0)=1) -> (substring before match=w119:string)  [unwired: 2 out]
              n66 = Search/Split String(string=w98, search string/char (-)=",") -> (substring before match=w100:string, match + rest of string=w102:string)  [unwired: 1 in, 1 out]
              n67 = Search/Split String(string=w102, search string/char (-)=",", offset (0)=1) -> (substring before match=w104:string, match + rest of string=w108:string)  [unwired: 1 out]
              n68 = Search/Split String(string=w108, search string/char (-)=",", offset (0)=1) -> (substring before match=w105:string)  [unwired: 2 out]
              n69 = call <vilib>:"Derivative x(t).vi"("X"=w80) -> ("dX/dt"=w79:dbl[])  [unwired: 9 in, 1 out]
              n70 = for {
                N: 3 -> [_]
                shift-right: [w249] -> _
                shift-left: w192 -> [w251]
                tunnel: [w247] -> w188 mode=indexing
                n71 = Search/Split String(string=w251, search string/char (-)="\t", offset (0)=1) -> (substring before match=w247:string, match + rest of string=w249:string)  [unwired: 1 out]
              }
              n72 = call "MARS3D Experiment Time.vi"("Time Experiment"=w87, "Time Calibration"=w88) -> ("Time elapsed (MIN)"=w86:dbl)  [unwired: 9 in]
              n73 = String Subset(string=w178, offset (0)=2) -> (substring=w84:string)  [unwired: 1 in]
              n74 = Negate(x=w79) -> (-x=w76:dbl[])
              n75 = String Subset(string=w160, offset (0)=2) -> (substring=w151:string)  [unwired: 1 in]
              n76 = String Subset(string=w148, offset (0)=2, length (rest)=3 ("length (rest)")) -> (substring=w144:string)
              n77 = String Subset(string=w153, offset (0)=2) -> (substring=w150:string)  [unwired: 1 in]
              n78 = String Subset(string=w140, offset (0)=2) -> (substring=w138:string)  [unwired: 1 in]
              n79 = Decimal String To Number(string=w173, offset=1) -> (number=w168:i32)  [unwired: 1 in, 1 out]
              n80 = Decimal String To Number(string=w137, offset=2) -> (number=w132:i32)  [unwired: 1 in, 1 out]
              n81 = call <vilib>:"Threshold Detector.vi"("width"=1, "threshold"=100.0, "X"=w76) -> ("Indices"=w75:i32[])  [unwired: 2 out]
              n82 = Decimal String To Number(string=w120, offset=1) -> (number=w114:i32)  [unwired: 1 in, 1 out]
              n83 = Decimal String To Number(string=w119, offset=1) -> (number=w113:i32)  [unwired: 1 in, 1 out]
              n84 = Decimal String To Number(string=w124, offset=2) -> (number=w115:i32)  [unwired: 1 in, 1 out]
              n85 = Decimal String To Number(string=w104, offset=1) -> (number=w92:i32)  [unwired: 1 in, 1 out]
              n86 = Decimal String To Number(string=w105, offset=1) -> (number=w91:i32)  [unwired: 1 in, 1 out]
              n87 = Decimal String To Number(string=w100, offset=2) -> (number=w93:i32)  [unwired: 1 in, 1 out]
              n88 = Index Array(array=w75) -> (element=w74:i32)  [unwired: 1 in]
              n89 = Match Pattern(string=w68, regular expression="<CAMERA ORIENTATION: *") -> (after substring=w70:string)  [unwired: 1 in, 3 out]
              n90 = case shown="True" "Automatic Calibration" {
                tunnel: w115 -> [_ w243]
                tunnel: w114 -> [_ w242]
                tunnel: w113 -> [_ w241]
                tunnel: w93 -> [_ w238]
                tunnel: w92 -> [_ w237]
                tunnel: w91 -> [_ w236]
                frame False {
                }
                frame True {
                  n91 = local read "Left Eye"() -> (w239:T5)
                  n92 = local read "Right Eye"() -> (w245:T5)
                  n93 = call "Mars3D calibration check.vi"("Numeric 3"=w238, "Right Eye in"=w245, "Numeric 2"=w237, "Numeric 6"=w243, "Left Eye in"=w239, "Numeric"=w236, "Numeric 4"=w241, "Numeric 5"=w242) -> ("no calibration"=w235:bool, "Left Eye out"=w240:T5, "Right Eye out"=w244:T5)  [unwired: 1 in]
                  n94 = case shown="True" w235 {
                    frame False {
                    }
                    frame True {
                      n95 = disable-structure shown="Disabled" {
                        frame Disabled {
                          n96 = local write "Automatic Calibration"(FALSE ("Automatic Calibration")) -> ()
                        }
                        frame Enabled {
                        }
                      }
                    }
                  }
                  n97 = local write "Right Eye"(w244) -> ()
                  n98 = local write "Left Eye"(w240) -> ()
                }
              }
              n99 = Match Pattern(string=w70, regular expression=">") -> (before substring=w67:string)  [unwired: 1 in, 3 out]
              n100 = case shown="\"STEP\", Default" w84 {
                tunnel: w83 -> [w223 w227]
                tunnel: [0.0 w226] -> w82
                tunnel: [w222 0] -> w81
                frame "STEP", Default {
                  n101 = Decimal String To Number(string=w223, offset=2 ("offset (0)")) -> (number=w222:i32)  [unwired: 1 in, 1 out]
                }
                frame "SINE" {
                  n102 = Fract/Exp String To Number(string=w227, offset=2) -> (number=w226:dbl)  [unwired: 2 in, 1 out]
                }
              }
              n103 = Bundle By Name(cluster=w164, "Experiment Parameters.Freq"=w82, "Experiment Parameters.Vel"=w168, "Experiment Parameters.Acc"=w81, "Experiment Parameters.Stimulus"=w84, "Parameter Time Series"="Plot Selection", "Parameter Impuls Series"="Plot Selection 2", "Experiment Parameters 2.Subject"=w151, "Experiment Parameters 2.Strain"=w150, "Experiment Parameters 2.Rotation plane"=w144, "Experiment Parameters 2.Experimenter"=w138, "Experiment Parameters 2.Trial"=w132, "Experiment Parameters 2.Time"=w86) -> (w165:T1)
              n104 = Strip Path(path=w182) -> (stripped path=w163:path, name=w162:string)
              n105 = case shown="\"Horizontal\", Default" w67 {
                tunnel: [enum16{"Horizontal", "Vertical"}."Horizontal" ("Stored Camera Orientation") enum16{"Horizontal", "Vertical"}."Vertical" ("Stored Camera Orientation")] -> w66
                frame "Horizontal", Default {
                  # "Cameras were selected as horizontally orientated.\nIf not specified this is the deault case as vertcial camera orientation did not exist."
                }
                frame "Vertical" {
                  # "Cameras were selected as vertically orientated."
                }
              }
              n106 = Insert Into Array(array=string[] ["Global Trigger"], new element=w188) -> (w189:string[])  [unwired: 1 in]
            }
            frame True {
              n107 = local write "stop 2"(TRUE ("stop 2")) -> ()
            }
          }
        }
        frame True {
        }
      }
    }
    frame #2 {
      n108 = local read "stop 2"() -> (w260:bool)
      n109 = case shown="False" w260 {
        tunnel: ["Angles" _] -> w266
        tunnel: [string[] ["Lx Position-in-Head", "Ly Position-in-Head", "Lz Position-in-Head", "Lx Velocity-in-Head", "Ly Velocity-in-Head", "Lz Velocity-in-Head", "Ll Velocity-in-Head", "Lr Velocity-in-Head", "Lx Accel-in-Head", "Ly Accel-in-Head", "Lz Accel-in-Head"] _] -> w265
        tunnel: w264 -> [w294 _]
        tunnel: w263 -> [w291 _]
        tunnel: [w311 _] -> w262
        tunnel: w261 -> [w296 _]
        tunnel: w259 -> [w293 _]
        tunnel: [w292 _] -> w258
        tunnel: w257 -> [w267 _]
        frame False {
          n110 = local read "Rev Cam?"() -> (w269:bool)
          n111 = Index Array(array=w296, index (col)=19 ("index (row)")) -> (element=w321:dbl[])  [unwired: 1 in]
          n112 = Index Array(array=w296, index (col)=20 ("index (row)")) -> (element=w320:dbl[])  [unwired: 1 in]
          n113 = Index Array(array=w296, index (col)=21 ("index (row)")) -> (element=w319:dbl[])  [unwired: 1 in]
          n114 = Index Array(array=w296, index (col)=0 ("index (row)")) -> (element=w313:dbl[])  [unwired: 1 in]
          n115 = Index Array(array=w296, index (col)=13 ("index (row)")) -> (element=w283:dbl[])  [unwired: 1 in]
          n116 = Index Array(array=w296, index (col)=14 ("index (row)")) -> (element=w282:dbl[])  [unwired: 1 in]
          n117 = Index Array(array=w296, index (col)=15 ("index (row)")) -> (element=w281:dbl[])  [unwired: 1 in]
          n118 = Index Array(array=w296, index (col)=16 ("index (row)")) -> (element=w280:dbl[])  [unwired: 1 in]
          n119 = Index Array(array=w296, index (col)=17 ("index (row)")) -> (element=w279:dbl[])  [unwired: 1 in]
          n120 = Index Array(array=w296, index (col)=18 ("index (row)")) -> (element=w278:dbl[])  [unwired: 1 in]
          n121 = call "Reverse Camera Orientation.vi"("P1X"=w283, "P1Y"=w282, "P2X"=w281, "P2Y"=w280, "P3X"=w279, "P3Y"=w278, "Apply Transform?"=w269, "Calibration Data"="Left Eye", "Stored Camera Orientation"=w267, "Eye"=enum16{"Right", "Left"}."Left") -> ("Calibration Data out"=w270:T5, "P1X out"=w277:dbl[], "P1Y out"=w276:dbl[], "P2X out"=w275:dbl[], "P2Y out"=w274:dbl[], "P3X out"=w273:dbl[], "P3Y out"=w272:dbl[])  [unwired: 3 in]
          n122 = Unbundle By Name(w270) -> ("y"=w304:dbl, "z"=w303:dbl)
          n123 = Subtract(x=w277, y=w304) -> (x-y=w310:dbl[])
          n124 = Subtract(x=w276, y=w303) -> (x-y=w309:dbl[])
          n125 = Subtract(x=w275, y=w304) -> (x-y=w308:dbl[])
          n126 = Subtract(x=w274, y=w303) -> (x-y=w307:dbl[])
          n127 = Subtract(x=w273, y=w304) -> (x-y=w306:dbl[])
          n128 = Subtract(x=w272, y=w303) -> (x-y=w305:dbl[])
          n129 = Build Array(w306, w305) -> (w332:dbl[][])
          n130 = Build Array(w308, w307) -> (w301:dbl[][])
          n131 = Build Array(w310, w309) -> (w302:dbl[][])
          n132 = Transpose 2D Array(2D array=w302) -> (transposed array=w318:dbl[][])
          n133 = Transpose 2D Array(2D array=w301) -> (transposed array=w317:dbl[][])
          n134 = Transpose 2D Array(2D array=w332) -> (transposed array=w316:dbl[][])
          n135 = local read "File"() -> (w287:path)
          n136 = Divide(x=w313, y=1000) -> (x/y=w298:dbl[])
          n137 = Empty String/Path?(string/path=w287) -> (empty?=w286:bool)
          n138 = Not(x=w286) -> (.not. x?=w285:bool)
          n139 = local read "Position Convention"() -> (w300:u16)
          n140 = case shown="False" "Savgol" {
            tunnel: w291 -> [_ w334]
            tunnel: [0 w334] -> w290
            frame False {
            }
            frame True {
            }
          }
          n141 = call "Process each eye.vi"("Camera coordinates rel to head co-ordinates"=w270, "Time (sec)"=w298, "Dir"=enum16{"Right", "Left"}."Left", "Hor (F)"=w321, "Ver (F)"=w320, "Posn, Vel, Acc 2"=w294, "Angles"="Angles", "Point1"=w318, "Trigger Edge"=w293, "Tor (F)"=w319, "Position Convention"=w300, "Point2"=w317, "Sample Rate"=w290, "Point3"=w316, "Savol Filter in percent"="Savol Filter in percent", "Use Last"=w285, "VOG system"="VOG system") -> ("Posn, Vel, Acc"=w312:dbl[][], "cancelled"=w292:bool)  [unwired: 1 in]
          n142 = case shown="True" TRUE ("Boolean") {
            tunnel: w294 -> [w342 _]
            tunnel: w298 -> [w341 _]
            tunnel: w312 -> [w340 w347]
            tunnel: w291 -> [w337 _]
            tunnel: [w335 w347] -> w311
            frame False {
              n143 = Array Size(array=w342) -> (size(s)=w346:i32[])
              n144 = Array Size(array=w340) -> (size(s)=w345:i32[])
              n145 = Index Array(array=w345, index=0) -> (element=w339:i32)
              n146 = Index Array(array=w346, index=1) -> (element=w338:i32)
              n147 = call "Interpolate Main.vi"("Length"=w338, "Data Channels"=w339, "NaN"=TRUE, "Sample Rate"=w337, "Data"=w340, "Time"=w341) -> ("Interp Data"=w335:dbl[][])  [unwired: 4 in]
            }
            frame True {
            }
          }
        }
        frame True {
        }
      }
    }
    frame #3 {
      n148 = local read "Rev Cam?"() -> (w349:bool)
      n149 = local read "stop 2"() -> (w353:bool)
      n150 = case shown="False" w353 {
        tunnel: w364 -> [w418 _]
        tunnel: w363 -> [w417 _]
        tunnel: w362 -> [w416 _]
        tunnel: w361 -> [w415 _]
        tunnel: [w413 _] -> w360
        tunnel: [w412 _] -> w359
        tunnel: w358 -> [w411 _]
        tunnel: w357 -> [w388 _]
        tunnel: w356 -> [w392 _]
        tunnel: w355 -> [w394 _]
        tunnel: w354 -> [w393 _]
        tunnel: w352 -> [w391 _]
        tunnel: [w390 _] -> w351
        tunnel: w350 -> [w366 _]
        tunnel: w349 -> [w367 _]
        tunnel: enum16{"Right", "Left"}."Right" ("Eye") -> [w365 _]
        frame False {
          n151 = Index Array(array=w418, index (col)=3 ("index (row)")) -> (element=w381:dbl[])  [unwired: 1 in]
          n152 = Index Array(array=w418, index (col)=4 ("index (row)")) -> (element=w380:dbl[])  [unwired: 1 in]
          n153 = Index Array(array=w418, index (col)=5 ("index (row)")) -> (element=w379:dbl[])  [unwired: 1 in]
          n154 = Index Array(array=w418, index (col)=6 ("index (row)")) -> (element=w378:dbl[])  [unwired: 1 in]
          n155 = Index Array(array=w418, index (col)=7 ("index (row)")) -> (element=w377:dbl[])  [unwired: 1 in]
          n156 = Index Array(array=w418, index (col)=8 ("index (row)")) -> (element=w376:dbl[])  [unwired: 1 in]
          n157 = Index Array(array=w418, index (col)=9 ("index (row)")) -> (element=w424:dbl[])  [unwired: 1 in]
          n158 = Index Array(array=w418, index (col)=10 ("index (row)")) -> (element=w423:dbl[])  [unwired: 1 in]
          n159 = Index Array(array=w418, index (col)=11 ("index (row)")) -> (element=w422:dbl[])  [unwired: 1 in]
          n160 = Index Array(array=w418, index (col)=0 ("index (row)")) -> (element=w397:dbl[])  [unwired: 1 in]
          n161 = call "Reverse Camera Orientation.vi"("P1X"=w381, "P1Y"=w380, "P2X"=w379, "P2Y"=w378, "P3X"=w377, "P3Y"=w376, "Apply Transform?"=w367, "Calibration Data"="Right Eye", "Stored Camera Orientation"=w366, "Eye"=w365) -> ("Calibration Data out"=w374:T5, "P1X out"=w373:dbl[], "P1Y out"=w372:dbl[], "P2X out"=w371:dbl[], "P2Y out"=w370:dbl[], "P3X out"=w369:dbl[], "P3Y out"=w368:dbl[])  [unwired: 3 in]
          n162 = Unbundle By Name(w374) -> ("y"=w402:dbl, "z"=w401:dbl)
          n163 = Subtract(x=w373, y=w402) -> (x-y=w408:dbl[])
          n164 = Subtract(x=w372, y=w401) -> (x-y=w407:dbl[])
          n165 = Subtract(x=w371, y=w402) -> (x-y=w406:dbl[])
          n166 = Subtract(x=w370, y=w401) -> (x-y=w405:dbl[])
          n167 = Subtract(x=w369, y=w402) -> (x-y=w404:dbl[])
          n168 = Subtract(x=w368, y=w401) -> (x-y=w403:dbl[])
          n169 = Build Array(w404, w403) -> (w437:dbl[][])
          n170 = Build Array(w406, w405) -> (w436:dbl[][])
          n171 = Build Array(w408, w407) -> (w435:dbl[][])
          n172 = Divide(x=w397, y=1000) -> (x/y=w398:dbl[])
          n173 = Transpose 2D Array(2D array=w435) -> (transposed array=w421:dbl[][])
          n174 = Transpose 2D Array(2D array=w436) -> (transposed array=w420:dbl[][])
          n175 = Transpose 2D Array(2D array=w437) -> (transposed array=w419:dbl[][])
          n176 = local read "Savol Filter in percent"() -> (w382:dbl)
          n177 = local read "File"() -> (w385:path)
          n178 = local read "VOG system"() -> (w399:enum16{"Mouse", "Chinchilla"})
          n179 = Empty String/Path?(string/path=w385) -> (empty?=w384:bool)
          n180 = local read "Savgol"() -> (w389:bool)
          n181 = Not(x=w384) -> (.not. x?=w383:bool)
          n182 = case shown="False" w389 {
            tunnel: w388 -> [_ w439]
            tunnel: [0 w439] -> w387
            frame False {
            }
            frame True {
            }
          }
          n183 = call "Process each eye.vi"("Camera coordinates rel to head co-ordinates"=w374, "Time (sec)"=w398, "Dir"=enum16{"Right", "Left"}."Right", "Hor (F)"=w424, "Ver (F)"=w423, "Posn, Vel, Acc 2"=w392, "Angles"=w417, "Point1"=w421, "Trigger Edge"=w391, "Tor (F)"=w422, "Position Convention"="Position Convention", "Point2"=w420, "Sample Rate"=w387, "Point3"=w419, "Savol Filter in percent"=w382, "Use Last"=w383, "VOG system"=w399) -> ("Posn, Vel, Acc"=w410:dbl[][], "cancelled"=w390:bool)  [unwired: 1 in]
          n184 = case shown="False" TRUE {
            tunnel: w398 -> [w444 _]
            tunnel: w410 -> [w443 w452]
            tunnel: w388 -> [w442 _]
            tunnel: w392 -> [w441 _]
            tunnel: [w440 w452] -> w409
            frame False {
              n185 = Array Size(array=w441) -> (size(s)=w451:i32[])
              n186 = Array Size(array=w443) -> (size(s)=w450:i32[])
              n187 = Index Array(array=w450, index=0) -> (element=w447:i32)
              n188 = Index Array(array=w451, index=1) -> (element=w446:i32)
              n189 = call "Interpolate Main.vi"("Length"=w446, "Data Channels"=w447, "NaN"=TRUE, "Sample Rate"=w442, "Data"=w443, "Time"=w444) -> ("Interp Data"=w440:dbl[][])  [unwired: 4 in]
            }
            frame True {
            }
          }
          n190 = Build Array (concatenate)(w416, w415, string[] ["Rx Position-in-Head", "Ry Position-in-Head", "Rz Position-in-Head", "Rx Velocity-in-Head", "Ry Velocity-in-Head", "Rz Velocity-in-Head", "Rl Velocity-in-Head", "Rr Velocity-in-Head", "Rx Accel-in-Head", "Ry Accel-in-Head", "Rz Accel-in-Head"], w393) -> (w412:string[])
          n191 = Build Array (concatenate)(w392, w411, w409, w394) -> (w413:dbl[][])
        }
        frame True {
          n192 = local write "stop 2"(FALSE ("stop 2")) -> ()
          "stop 3" <- TRUE ("stop 3")
        }
      }
    }
    frame #4 {
      n193 = Unbundle By Name(w463) -> ("desaccading parameters"=w464:T7)
      n194 = local read "Impulse Plane 2"() -> (w460:T6)
      n195 = local read "Acc Range"() -> (w467:dbl)
      n196 = local read "Impulse dir"() -> (w466:bool)
      n197 = local read "Tolerance"() -> (w468:i32)
      n198 = And(x=w459, y=w458) -> (x .and. y?=w455:bool)
      n199 = Bundle(cluster=w464, "Tolerance"=w468, "Acc Range"=w467, "Sample Rate"=w465, "Impulse Plane 2"=w460, "Impulse dir"=w466) -> (w462:T7)
      n200 = Bundle By Name(cluster=w463, "desaccading parameters"=w462) -> (w461:T1)
      n201 = local read "stop 2"() -> (w457:bool)
      n202 = Or(x=w455, y=w457) -> (x .or. y?=w456:bool)
    }
  }
  n203 = case shown="False" w1 {
    tunnel: w10 -> [w476 _]
    tunnel: w9 -> [w475 _]
    tunnel: w7 -> [w474 _]
    tunnel: w6 -> [w473 _]
    tunnel: [w472 w477] -> w5
    tunnel: w4 -> [w470 _]
    tunnel: w3 -> [w469 _]
    tunnel: "Statemachine Data IN" -> [_ w477]
    frame False {
      n204 = Bundle(w475, w476, w474) -> (w471:cluster{dbl[][], i32, string[]})  [unwired: 1 in]
      n205 = Bundle By Name(cluster=w473, "filename"=w469, "Experiment data path"=w470, "Data File"=w471) -> (w472:T1)
    }
    frame True {
    }
  }
  "Statemachine Data OUT" <- w5
  n206 = Request Deallocation(TRUE ("flag")) -> ()
